vi "Plane_extraction.vi"() -> ()   [LabVIEW 2013]
uses:
  <vilib>/vision/NI_Vision_Development_Module.lvlib
panel:
  out "Blue":T1(plugin-control)
  out "Green":T1(plugin-control)
  out "Red":T1(plugin-control)
  in  "Color Mode":u16(ring) items=["RGB", "HSL", "HSV", "HSI"]
  in  "Path":path
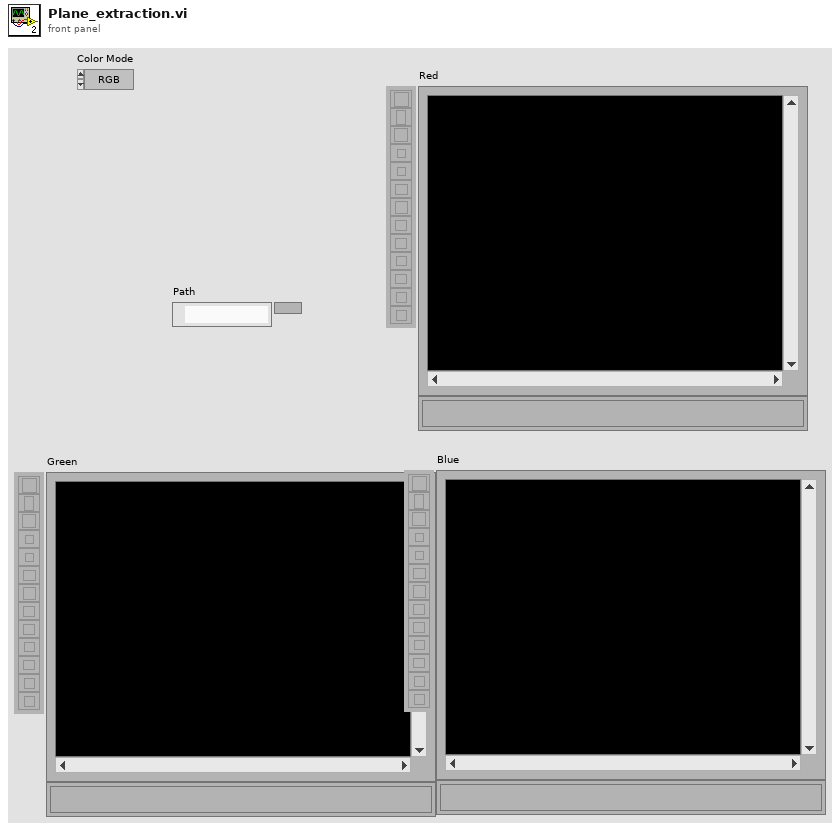
[diagram p1: front panel]
types:
  T1 = typedef "IMAQ Image.ctl" = refnum<image>
  T2 = typedef "Image Type" = u32
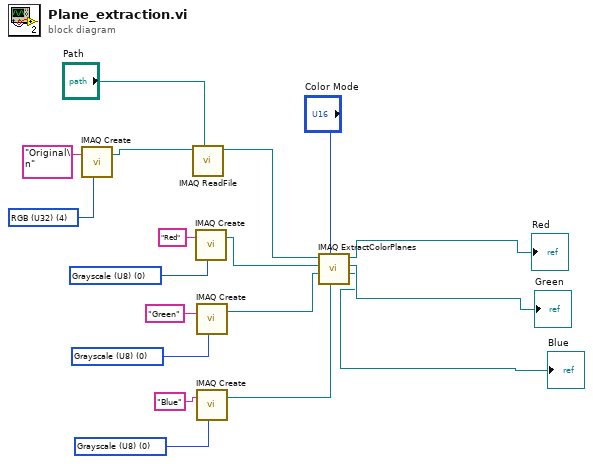
[diagram p0: block diagram]
diagram:
  w9 = T2 0 items=["Grayscale (U8)", "Grayscale (I16)", "Grayscale (SGL)", "Complex (CSG)", "RGB (U32)", "HSL (U32)", "RGB (U64)", "Grayscale (U16)"] ("Image Type")
  w10 = T2 0 items=["Grayscale (U8)", "Grayscale (I16)", "Grayscale (SGL)", "Complex (CSG)", "RGB (U32)", "HSL (U32)", "RGB (U64)", "Grayscale (U16)"] ("Image Type")
  w11 = T2 0 items=["Grayscale (U8)", "Grayscale (I16)", "Grayscale (SGL)", "Complex (CSG)", "RGB (U32)", "HSL (U32)", "RGB (U64)", "Grayscale (U16)"] ("Image Type")
  w12 = T2 4 items=["Grayscale (U8)", "Grayscale (I16)", "Grayscale (SGL)", "Complex (CSG)", "RGB (U32)", "HSL (U32)", "RGB (U64)", "Grayscale (U16)"] ("Image Type")
  n1 = call "IMAQ Create"("Image Name"="Original\n", "Image Type"=w12) -> ("New Image"=w14:T1)  [unwired: 3 in, 1 out]
  n2 = call "IMAQ ReadFile"("File Path"="Path", "Image"=w14) -> ("Image Out"=w8:T1)  [unwired: 5 in, 4 out]
  n3 = call "IMAQ Create"("Image Name"="Red", "Image Type"=w11) -> ("New Image"=w7:T1)  [unwired: 3 in, 1 out]
  n4 = call "IMAQ Create"("Image Name"="Green", "Image Type"=w10) -> ("New Image"=w6:T1)  [unwired: 3 in, 1 out]
  n5 = call "IMAQ Create"("Image Name"="Blue", "Image Type"=w9) -> ("New Image"=w5:T1)  [unwired: 3 in, 1 out]
  n6 = call "IMAQ ExtractColorPlanes"("Blue or Luma or Val or Inten Plane"=w5, "Color Mode"="Color Mode", "Green or Sat Plane"=w6, "Red or Hue Plane"=w7, "Image Src"=w8) -> ("Blue or Luma or Val or Inten Plane out"=→"Blue":T1, "Green or Sat Plane out"=→"Green":T1, "Red or Hue Plane out"=→"Red":T1)  [unwired: 3 in, 1 out]
